vi "Create 1bit bmp image.vi"(8 "error in (no error)":errorcluster, 11 "path to BMP file":path=path "M:/DigiLens-1276/Production Print Pattern App/DL2ExportedDitheredImages/20240327_C30v3_1_DL_2/12.bmp") -> (0 "error out":errorcluster)   [LabVIEW 2022 SP3]
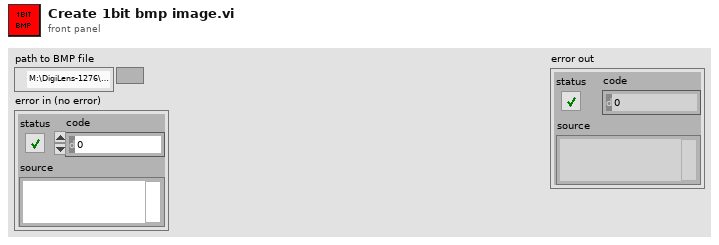
[diagram p1: front panel]
types:
  T1 = typedef "imagedata.ctl" = cluster{"image type":i32, "image depth":i32, "image":u8[], "mask":u8[], "colors":u32[], "Rectangle":cluster{"left":i16, "top":i16, "right":i16, "bottom":i16}}
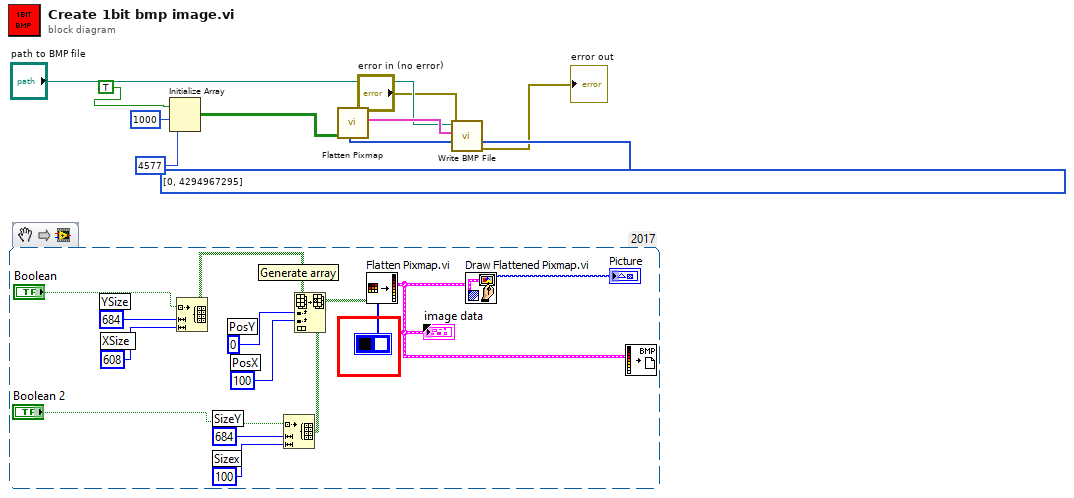
[diagram p0: block diagram]
diagram:
  n1 = Initialize Array(TRUE, 1000 ("dimension size"), 4577 ("dimension size")) -> (w5:bool[][])
  n2 = call <vilib>:"Flatten Pixmap.vi"("colors"=u32[] [0, 4294967295], "1-bit pixmap"=w5) -> ("image data"=w4:T1)  [unwired: 9 in]
  n3 = call <vilib>:"Write BMP File.vi"("error in (no error)"="error in (no error)", "image data"=w4, "path to BMP file"="path to BMP file") -> ("error out"=→"error out":errorcluster)  [unwired: 7 in, 1 out]
